vi "GeoData.vi"() -> ()   [LabVIEW 2017] (continued)
Niagara County\tH1\n14028\t36063\tBurt\tNY\tNiagara County\tH1\n14302\t36063\tNiagara falls\tNY\tNiagara County\tH1\n14032\t36063\tClarence center\tNY\tNiagara County\tH1\n14067\t36063\tGasport\tNY\tNiagara County\tH1\n14131\t36063\tRansomville\tNY\tNiagara County\tH1\n14008\t36063\tAppleton\tNY\tNiagara County\tH1\n14174\t36063\tYoungstown\tNY\tNiagara County\tH1\n14304\t36063\tNiagara falls\tNY\tNiagara County\tH1\n14012\t36063\tBarker\tNY\tNiagara County\tH1\n14108\t36063\tNewfane\tNY\tNiagara County\tH1\n14098\t36063\tLyndonville\tNY\tNiagara County\tH1\n14107\t36063\tModel city\tNY\tNiagara County\tH1\n14120\t36063\tNorth tonawanda\tNY\tNiagara County\tH1\n14001\t36063\tAkron\tNY\tNiagara County\tH1\n14092\t36063\tLewiston\tNY\tNiagara County\tH1\n14132\t36063\tSanborn\tNY\tNiagara County\tH1\n14303\t36063\tNiagara falls\tNY\tNiagara County\tH1\n14301\t36063\tNiagara falls\tNY\tNiagara County\tH1\n14305\t36063\tNiagara falls\tNY\tNiagara County\tH1\n14095\t36063\tLockport\tNY\tNiagara County\tH1\n14144\t36063\tStella niagara\tNY\tNiagara County\tH1\n13483\t36065\tWestdale\tNY\tOneida County\tH1\n13461\t36065\tSherrill\tNY\tOneida County\tH1\n13313\t36065\tBridgewater\tNY\tOneida County\tH1\n13301\t36065\tAlder creek\tNY\tOneida County\tH1\n13123\t36065\tNorth bay\tNY\tOneida County\tH1\n13338\t36065\tForestport\tNY\tOneida County\tH1\n13478\t36065\tVerona\tNY\tOneida County\tH1\n13354\t36065\tHolland patent\tNY\tOneida County\tH1\n13322\t36065\tClayville\tNY\tOneida County\tH1\n13486\t36065\tWesternville\tNY\tOneida County\tH1\n13032\t36065\tCanastota\tNY\tOneida County\tH1\n13308\t36065\tBlossvale\tNY\tOneida County\tH1\n13319\t36065\tChadwicks\tNY\tOneida County\tH1\n13413\t36065\tNew hartford\tNY\tOneida County\tH1\n13323\t36065\tClinton\tNY\tOneida County\tH1\n13501\t36065\tUtica\tNY\tOneida County\tH1\n13440\t36065\tRome\tNY\tOneida County\tH1\n13469\t36065\tStittville\tNY\tOneida County\tH1\n13441\t36065\tRome\tNY\tOneida County\tH1\n13162\t36065\tVerona beach\tNY\tOneida County\tH1\n13456\t36065\tSauquoit\tNY\tOneida County\tH1\n13495\t36065\tYorkville\tNY\tOneida County\tH1\n13424\t36065\tOriskany\tNY\tOneida County\tH1\n13362\t36065\tKnoxboro\tNY\tOneida County\tH1\n13304\t36065\tBarneveld\tNY\tOneida County\tH1\n13303\t36065\tAva\tNY\tOneida County\tH1\n13403\t36065\tMarcy\tNY\tOneida County\tH1\n13438\t36065\tRemsen\tNY\tOneida County\tH1\n13491\t36065\tWest winfield\tNY\tOneida County\tH1\n13417\t36065\tNew york mills\tNY\tOneida County\tH1\n13431\t36065\tPoland\tNY\tOneida County\tH1\n13435\t36065\tProspect\tNY\tOneida County\tH1\n13341\t36065\tFranklin springs\tNY\tOneida County\tH1\n13318\t36065\tCassville\tNY\tOneida County\tH1\n13409\t36065\tMunnsville\tNY\tOneida County\tH1\n13471\t36065\tTaberg\tNY\tOneida County\tH1\n13502\t36065\tUtica\tNY\tOneida County\tH1\n13490\t36065\tWestmoreland\tNY\tOneida County\tH1\n13321\t36065\tClark mills\tNY\tOneida County\tH1\n13401\t36065\tMc connellsville\tNY\tOneida County\tH1\n13042\t36065\tCleveland\tNY\tOneida County\tH1\n13309\t36065\tBoonville\tNY\tOneida County\tH1\n13316\t36065\tCamden\tNY\tOneida County\tH1\n13402\t36065\tMadison\tNY\tOneida County\tH1\n13476\t36065\tVernon\tNY\tOneida County\tH1\n13480\t36065\tWaterville\tNY\tOneida County\tH1\n13425\t36065\tOriskany falls\tNY\tOneida County\tH1\n13477\t36065\tVernon center\tNY\tOneida County\tH1\n13421\t36065\tOneida\tNY\tOneida County\tH1\n13492\t36065\tWhitesboro\tNY\tOneida County\tH1\n13489\t36065\tWest leyden\tNY\tOneida County\tH1\n13054\t36065\tDurhamville\tNY\tOneida County\tH1\n13157\t36065\tSylvan beach\tNY\tOneida County\tH1\n13363\t36065\tLee center\tNY\tOneida County\tH1\n13494\t36065\tWoodgate\tNY\tOneida County\tH1\n13328\t36065\tDeansboro\tNY\tOneida County\tH1\n13352\t36065\tHinckley\tNY\tOneida County\tH1\n13455\t36065\tSangerfield\tNY\tOneida County\tH1\n13479\t36065\tWashington mills\tNY\tOneida County\tH1\n13504\t36065\tUtica\tNY\tOneida County\tH1\n13035\t36067\tCazenovia\tNY\tOnondaga County\tH1\n13036\t36067\tCentral square\tNY\tOnondaga County\tH1\n13166\t36067\tWeedsport\tNY\tOnondaga County\tH1\n13020\t36067\tApulia station\tNY\tOnondaga County\tH1\n13120\t36067\tNedrow\tNY\tOnondaga County\tH1\n13206\t36067\tSyracuse\tNY\tOnondaga County\tH1\n13207\t36067\tSyracuse\tNY\tOnondaga County\tH1\n13244\t36067\tSyracuse\tNY\tOnondaga County\tH1\n13218\t36067\tSyracuse\tNY\tOnondaga County\tH1\n13290\t36067\tSyracuse\tNY\tOnondaga County\tH1\n13031\t36067\tCamillus\tNY\tOnondaga County\tH1\n13027\t36067\tBaldwinsville\tNY\tOnondaga County\tH1\n13069\t36067\tFulton\tNY\tOnondaga County\tH1\n13090\t36067\tLiverpool\tNY\tOnondaga County\tH1\n13152\t36067\tSkaneateles\tNY\tOnondaga County\tH1\n13112\t36067\tMemphis\tNY\tOnondaga County\tH1\n13030\t36067\tBridgeport\tNY\tOnondaga County\tH1\n13141\t36067\tPreble\tNY\tOnondaga County\tH1\n13153\t36067\tSkaneateles falls\tNY\tOnondaga County\tH1\n13029\t36067\tBrewerton\tNY\tOnondaga County\tH1\n13033\t36067\tCato\tNY\tOnondaga County\tH1\n13084\t36067\tLa fayette\tNY\tOnondaga County\tH1\n13080\t36067\tJordan\tNY\tOnondaga County\tH1\n13110\t36067\tMarietta\tNY\tOnondaga County\tH1\n13219\t36067\tSyracuse\tNY\tOnondaga County\tH1\n13224\t36067\tSyracuse\tNY\tOnondaga County\tH1\n13210\t36067\tSyracuse\tNY\tOnondaga County\tH1\n13235\t36067\tSyracuse\tNY\tOnondaga County\tH1\n13063\t36067\tFabius\tNY\tOnondaga County\tH1\n13217\t36067\tSyracuse\tNY\tOnondaga County\tH1\n13201\t36067\tSyracuse\tNY\tOnondaga County\tH1\n13225\t36067\tSyracuse\tNY\tOnondaga County\tH1\n13078\t36067\tJamesville\tNY\tOnondaga County\tH1\n13088\t36067\tLiverpool\tNY\tOnondaga County\tH1\n13077\t36067\tHomer\tNY\tOnondaga County\tH1\n13135\t36067\tPhoenix\tNY\tOnondaga County\tH1\n13108\t36067\tMarcellus\tNY\tOnondaga County\tH1\n13122\t36067\tNew woodstock\tNY\tOnondaga County\tH1\n13214\t36067\tSyracuse\tNY\tOnondaga County\tH1\n13215\t36067\tSyracuse\tNY\tOnondaga County\tH1\n13212\t36067\tSyracuse\tNY\tOnondaga County\tH1\n13204\t36067\tSyracuse\tNY\tOnondaga County\tH1\n13261\t36067\tSyracuse\tNY\tOnondaga County\tH1\n13039\t36067\tCicero\tNY\tOnondaga County\tH1\n13037\t36067\tChittenango\tNY\tOnondaga County\tH1\n13104\t36067\tManlius\tNY\tOnondaga County\tH1\n13057\t36067\tEast syracuse\tNY\tOnondaga County\tH1\n13052\t36067\tDe ruyter\tNY\tOnondaga County\tH1\n13060\t36067\tElbridge\tNY\tOnondaga County\tH1\n13205\t36067\tSyracuse\tNY\tOnondaga County\tH1\n13089\t36067\tLiverpool\tNY\tOnondaga County\tH1\n13138\t36067\tPompey\tNY\tOnondaga County\tH1\n13051\t36067\tDelphi falls\tNY\tOnondaga County\tH1\n13119\t36067\tMottville\tNY\tOnondaga County\tH1\n13252\t36067\tSyracuse\tNY\tOnondaga County\tH1\n13021\t36067\tAuburn\tNY\tOnondaga County\tH1\n13202\t36067\tSyracuse\tNY\tOnondaga County\tH1\n13203\t36067\tSyracuse\tNY\tOnondaga County\tH1\n13116\t36067\tMinoa\tNY\tOnondaga County\tH1\n13137\t36067\tPlainville\tNY\tOnondaga County\tH1\n13082\t36067\tKirkville\tNY\tOnondaga County\tH1\n13066\t36067\tFayetteville\tNY\tOnondaga County\tH1\n13158\t36067\tTruxton\tNY\tOnondaga County\tH1\n13159\t36067\tTully\tNY\tOnondaga County\tH1\n13164\t36067\tWarners\tNY\tOnondaga County\tH1\n13208\t36067\tSyracuse\tNY\tOnondaga County\tH1\n13211\t36067\tSyracuse\tNY\tOnondaga County\tH1\n13209\t36067\tSyracuse\tNY\tOnondaga County\tH1\n13220\t36067\tSyracuse\tNY\tOnondaga County\tH1\n13041\t36067\tClay\tNY\tOnondaga County\tH1\n14512\t36069\tNaples\tNY\tOntario County\tH1\n14585\t36069\tWest bloomfield\tNY\tOntario County\tH1\n14534\t36069\tPittsford\tNY\tOntario County\tH1\n14472\t36069\tHoneoye falls\tNY\tOntario County\tH1\n14544\t36069\tRushville\tNY\tOntario County\tH1\n14425\t36069\tFarmington\tNY\tOntario County\tH1\n14463\t36069\tHall\tNY\tOntario County\tH1\n14475\t36069\tIonia\tNY\tOntario County\tH1\n14547\t36069\tSeneca castle\tNY\tOntario County\tH1\n14560\t36069\tSpringwater\tNY\tOntario County\tH1\n14424\t36069\tCanandaigua\tNY\tOntario County\tH1\n14504\t36069\tManchester\tNY\tOntario County\tH1\n14537\t36069\tPort gibson\tNY\tOntario County\tH1\n14485\t36069\tLima\tNY\tOntario County\tH1\n14487\t36069\tLivonia\tNY\tOntario County\tH1\n14513\t36069\tNewark\tNY\tOntario County\tH1\n14564\t36069\tVictor\tNY\tOntario County\tH1\n14561\t36069\tStanley\tNY\tOntario County\tH1\n14466\t36069\tHemlock\tNY\tOntario County\tH1\n14461\t36069\tGorham\tNY\tOntario County\tH1\n14432\t36069\tClifton springs\tNY\tOntario County\tH1\n14489\t36069\tLyons\tNY\tOntario County\tH1\n14456\t36069\tGeneva\tNY\tOntario County\tH1\n14471\t36069\tHoneoye\tNY\tOntario County\tH1\n14522\t36069\tPalmyra\tNY\tOntario County\tH1\n14548\t36069\tShortsville\tNY\tOntario County\tH1\n14453\t36069\tFishers\tNY\tOntario County\tH1\n14518\t36069\tOaks corners\tNY\tOntario County\tH1\n14469\t36069\tBloomfield\tNY\tOntario County\tH1\n14532\t36069\tPhelps\tNY\tOntario County\tH1\n10924\t36071\tGoshen\tNY\tOrange County\tH1\n10987\t36071\tTuxedo park\tNY\tOrange County\tH1\n12520\t36071\tCornwall on hudson\tNY\tOrange County\tH1\n12553\t36071\tNew windsor\tNY\tOrange County\tH1\n12566\t36071\tPine bush\tNY\tOrange County\tH1\n12589\t36071\tWallkill\tNY\tOrange County\tH1\n12575\t36071\tRock tavern\tNY\tOrange County\tH1\n12785\t36071\tWestbrookville\tNY\tOrange County\tH1\n10910\t36071\tArden\tNY\tOrange County\tH1\n10918\t36071\tChester\tNY\tOrange County\tH1\n12543\t36071\tMaybrook\tNY\tOrange County\tH1\n12586\t36071\tWalden\tNY\tOrange County\tH1\n10933\t36071\tJohnson\tNY\tOrange County\tH1\n10981\t36071\tSugar loaf\tNY\tOrange County\tH1\n10979\t36071\tSterling forest\tNY\tOrange County\tH1\n10959\t36071\tNew milford\tNY\tOrange County\tH1\n10925\t36071\tGreenwood lake\tNY\tOrange County\tH1\n10958\t36071\tNew hampton\tNY\tOrange County\tH1\n10985\t36071\tThompson ridge\tNY\tOrange County\tH1\n12518\t36071\tCornwall\tNY\tOrange County\tH1\n10928\t36071\tHighland falls\tNY\tOrange County\tH1\n10919\t36071\tCircleville\tNY\tOrange County\tH1\n12551\t36071\tNewburgh\tNY\tOrange County\tH1\n12584\t36071\tVails gate\tNY\tOrange County\tH1\n10953\t36071\tMountainville\tNY\tOrange County\tH1\n10914\t36071\tBlooming grove\tNY\tOrange County\tH1\n12549\t36071\tMontgomery\tNY\tOrange County\tH1\n12577\t36071\tSalisbury mills\tNY\tOrange County\tH1\n12729\t36071\tCuddebackville\tNY\tOrange County\tH1\n10932\t36071\tHowells\tNY\tOrange County\tH1\n10917\t36071\tCentral valley\tNY\tOrange County\tH1\n10926\t36071\tHarriman\tNY\tOrange County\tH1\n10998\t36071\tWesttown\tNY\tOrange County\tH1\n12542\t36071\tMarlboro\tNY\tOrange County\tH1\n12721\t36071\tBloomingburg\tNY\tOrange County\tH1\n10916\t36071\tCampbell hall\tNY\tOrange County\tH1\n10988\t36071\tUnionville\tNY\tOrange County\tH1\n10975\t36071\tSouthfields\tNY\tOrange County\tH1\n10940\t36071\tMiddletown\tNY\tOrange County\tH1\n10950\t36071\tMonroe\tNY\tOrange County\tH1\n12754\t36071\tLiberty\tNY\tOrange County\tH1\n10912\t36071\tBellvale\tNY\tOrange County\tH1\n10915\t36071\tBullville\tNY\tOrange County\tH1\n10941\t36071\tMiddletown\tNY\tOrange County\tH1\n10930\t36071\tHighland mills\tNY\tOrange County\tH1\n10990\t36071\tWarwick\tNY\tOrange County\tH1\n10973\t36071\tSlate hill\tNY\tOrange County\tH1\n10969\t36071\tPine island\tNY\tOrange County\tH1\n10996\t36071\tWest point\tNY\tOrange County\tH1\n12771\t36071\tPort jervis\tNY\tOrange County\tH1\n12552\t36071\tNewburgh\tNY\tOrange County\tH1\n12555\t36071\tNewburgh\tNY\tOrange County\tH1\n10921\t36071\tFlorida\tNY\tOrange County\tH1\n10963\t36071\tOtisville\tNY\tOrange County\tH1\n10992\t36071\tWashingtonville\tNY\tOrange County\tH1\n12550\t36071\tNewburgh\tNY\tOrange County\tH1\n12780\t36071\tSparrow bush\tNY\tOrange County\tH1\n10949\t36071\tMonroe\tNY\tOrange County\tH1\n12746\t36071\tHuguenot\tNY\tOrange County\tH1\n10922\t36071\tFort montgomery\tNY\tOrange County\tH1\n14464\t36073\tHamlin\tNY\tOrleans County\tH1\n14476\t36073\tKendall\tNY\tOrleans County\tH1\n14452\t36073\tFancher\tNY\tOrleans County\tH1\n14105\t36073\tMiddleport\tNY\tOrleans County\tH1\n14420\t36073\tBrockport\tNY\tOrleans County\tH1\n14416\t36073\tBergen\tNY\tOrleans County\tH1\n14058\t36073\tElba\tNY\tOrleans County\tH1\n14422\t36073\tByron\tNY\tOrleans County\tH1\n14429\t36073\tClarendon\tNY\tOrleans County\tH1\n14012\t36073\tBarker\tNY\tOrleans County\tH1\n14103\t36073\tMedina\tNY\tOrleans County\tH1\n14098\t36073\tLyndonville\tNY\tOrleans County\tH1\n14477\t36073\tKent\tNY\tOrleans County\tH1\n14125\t36073\tOakfield\tNY\tOrleans County\tH1\n14411\t36073\tAlbion\tNY\tOrleans County\tH1\n14470\t36073\tHolley\tNY\tOrleans County\tH1\n14571\t36073\tWaterport\tNY\tOrleans County\tH1\n14479\t36073\tKnowlesville\tNY\tOrleans County\tH1\n13036\t36075\tCentral square\tNY\tOswego County\tH1\n13074\t36075\tHannibal\tNY\tOswego County\tH1\n13111\t36075\tMartville\tNY\tOswego County\tH1\n13145\t36075\tSandy creek\tNY\tOswego County\tH1\n13302\t36075\tAltmar\tNY\tOswego County\tH1\n13483\t36075\tWestdale\tNY\tOswego County\tH1\n13144\t36075\tRichland\tNY\tOswego County\tH1\n13167\t36075\tWest monroe\tNY\tOswego County\tH1\n13132\t36075\tPennellville\tNY\tOswego County\tH1\n13069\t36075\tFulton\tNY\tOswego County\tH1\n13121\t36075\tNew haven\tNY\tOswego County\tH1\n13033\t36075\tCato\tNY\tOswego County\tH1\n13493\t36075\tWilliamstown\tNY\tOswego County\tH1\n13661\t36075\tMannsville\tNY\tOswego County\tH1\n13426\t36075\tOrwell\tNY\tOswego County\tH1\n13093\t36075\tLycoming\tNY\tOswego County\tH1\n13044\t36075\tConstantia\tNY\tOswego County\tH1\n13142\t36075\tPulaski\tNY\tOswego County\tH1\n13135\t36075\tPhoenix\tNY\tOswego County\tH1\n13103\t36075\tMallory\tNY\tOswego County\tH1\n13437\t36075\tRedfield\tNY\tOswego County\tH1\n13126\t36075\tOswego\tNY\tOswego County\tH1\n13042\t36075\tCleveland\tNY\tOswego County\tH1\n13156\t36075\tSterling\tNY\tOswego County\tH1\n13316\t36075\tCamden\tNY\tOswego County\tH1\n13076\t36075\tHastings\tNY\tOswego County\tH1\n13115\t36075\tMinetto\tNY\tOswego County\tH1\n13114\t36075\tMexico\tNY\tOswego County\tH1\n13131\t36075\tParish\tNY\tOswego County\tH1\n13028\t36075\tBernhards bay\tNY\tOswego County\tH1\n13083\t36075\tLacona\tNY\tOswego County\tH1\n12155\t36077\tSchenevus\tNY\tOtsego County\tH1\n13796\t36077\tLaurens\tNY\tOtsego County\tH1\n13315\t36077\tBurlington flats\tNY\tOtsego County\tH1\n13333\t36077\tEast springfield\tNY\tOtsego County\tH1\n13457\t36077\tSchuyler lake\tNY\tOtsego County\tH1\n12149\t36077\tRichmondville\tNY\tOtsego County\tH1\n13320\t36077\tCherry valley\tNY\tOtsego County\tH1\n13450\t36077\tRoseboom\tNY\tOtsego County\tH1\n13834\t36077\tPortlandville\tNY\tOtsego County\tH1\n13459\t36077\tSharon springs\tNY\tOtsego County\tH1\n13849\t36077\tUnadilla\tNY\tOtsego County\tH1\n13361\t36077\tJordanville\tNY\tOtsego County\tH1\n13482\t36077\tWest burlington\tNY\tOtsego County\tH1\n13415\t36077\tNew lisbon\tNY\tOtsego County\tH1\n12036\t36077\tCharlotteville\tNY\tOtsego County\tH1\n13335\t36077\tEdmeston\tNY\tOtsego County\tH1\n13809\t36077\tMount upton\tNY\tOtsego County\tH1\n13337\t36077\tFly creek\tNY\tOtsego County\tH1\n12043\t36077\tCobleskill\tNY\tOtsego County\tH1\n13348\t36077\tHartwick\tNY\tOtsego County\tH1\n13317\t36077\tCanajoharie\tNY\tOtsego County\tH1\n13411\t36077\tNew berlin\tNY\tOtsego County\tH1\n13491\t36077\tWest winfield\tNY\tOtsego County\tH1\n13485\t36077\tWest edmeston\tNY\tOtsego County\tH1\n13439\t36077\tRichfield springs\tNY\tOtsego County\tH1\n13733\t36077\tBainbridge\tNY\tOtsego County\tH1\n13810\t36077\tMount vision\tNY\tOtsego County\tH1\n13861\t36077\tWest oneonta\tNY\tOtsego County\tH1\n13825\t36077\tOtego\tNY\tOtsego County\tH1\n13488\t36077\tWestford\tNY\tOtsego County\tH1\n12064\t36077\tEast worcester\tNY\tOtsego County\tH1\n13747\t36077\tColliersville\tNY\tOtsego County\tH1\n13838\t36077\tSidney\tNY\tOtsego County\tH1\n13326\t36077\tCooperstown\tNY\tOtsego County\tH1\n13807\t36077\tMilford\tNY\tOtsego County\tH1\n13468\t36077\tSpringfield center\tNY\tOtsego County\tH1\n13750\t36077\tDavenport\tNY\tOtsego County\tH1\n13776\t36077\tGilbertsville\tNY\tOtsego County\tH1\n12116\t36077\tMaryland\tNY\tOtsego County\tH1\n12197\t36077\tWorcester\tNY\tOtsego County\tH1\n13820\t36077\tOneonta\tNY\tOtsego County\tH1\n13808\t36077\tMorris\tNY\tOtsego County\tH1\n13775\t36077\tFranklin\tNY\tOtsego County\tH1\n13843\t36077\tSouth new berlin\tNY\tOtsego County\tH1\n13859\t36077\tWells bridge\tNY\tOtsego County\tH1\n13342\t36077\tGarrattsville\tNY\tOtsego County\tH1\n12533\t36079\tHopewell junction\tNY\tPutnam County\tH1\n12563\t36079\tPatterson\tNY\tPutnam County\tH1\n10542\t36079\tMahopac falls\tNY\tPutnam County\tH1\n10512\t36079\tCarmel\tNY\tPutnam County\tH1\n10509\t36079\tBrewster\tNY\tPutnam County\tH1\n12564\t36079\tPawling\tNY\tPutnam County\tH1\n10505\t36079\tBaldwin place\tNY\tPutnam County\tH1\n10516\t36079\tCold spring\tNY\tPutnam County\tH1\n12531\t36079\tHolmes\tNY\tPutnam County\tH1\n10541\t36079\tMahopac\tNY\tPutnam County\tH1\n10579\t36079\tPutnam valley\tNY\tPutnam County\tH1\n12582\t36079\tStormville\tNY\tPutnam County\tH1\n10524\t36079\tGarrison\tNY\tPutnam County\tH1\n10588\t36079\tShrub oak\tNY\tPutnam County\tH1\n10567\t36079\tCortlandt manor\tNY\tPutnam County\tH1\n10598\t36079\tYorktown heights\tNY\tPutnam County\tH1\n12524\t36079\tFishkill\tNY\tPutnam County\tH1\n10537\t36079\tLake peekskill\tNY\tPutnam County\tH1\n11001\t36081\tFloral park\tNY\tQueens County\tH6\n11102\t36081\tAstoria\tNY\tQueens County\tH6\n11369\t36081\tEast elmhurst\tNY\tQueens County\tH6\n11418\t36081\tRichmond hill\tNY\tQueens County\tH6\n11420\t36081\tSouth ozone park\tNY\tQueens County\tH6\n11422\t36081\tRosedale\tNY\tQueens County\tH6\n11419\t36081\tSouth richmond hill\tNY\tQueens County\tH6\n11427\t36081\tQueens village\tNY\tQueens County\tH6\n11693\t36081\tFar rockaway\tNY\tQueens County\tH6\n11020\t36081\tGreat neck\tNY\tQueens County\tH6\n11106\t36081\tAstoria\tNY\tQueens County\tH6\n11354\t36081\tFlushing\tNY\tQueens County\tH6\n11368\t36081\tCorona\tNY\tQueens County\tH6\n11370\t36081\tEast elmhurst\tNY\tQueens County\tH6\n11372\t36081\tJackson heights\tNY\tQueens County\tH6\n11377\t36081\tWoodside\tNY\tQueens County\tH6\n11413\t36081\tSpringfield gardens\tNY\tQueens County\tH6\n11433\t36081\tJamaica\tNY\tQueens County\tH6\n11417\t36081\tOzone park\tNY\tQueens County\tH6\n11428\t36081\tQueens village\tNY\tQueens County\tH6\n11692\t36081\tArverne\tNY\tQueens County\tH6\n11371\t36081\tFlushing\tNY\tQueens County\tH6\n11359\t36081\tBayside\tNY\tQueens County\tH6\n11208\t36081\tBrooklyn\tNY\tQueens County\tH6\n11352\t36081\tFlushing\tNY\tQueens County\tH6\n11366\t36081\tFresh meadows\tNY\tQueens County\tH6\n11430\t36081\tJamaica\tNY\tQueens County\tH6\n11439\t36081\tJamaica\tNY\tQueens County\tH6\n11431\t36081\tJamaica\tNY\tQueens County\tH6\n11405\t36081\tJamaica\tNY\tQueens County\tH6\n11105\t36081\tAstoria\tNY\tQueens County\tH6\n11109\t36081\tLong island city\tNY\tQueens County\tH6\n11367\t36081\tFlushing\tNY\tQueens County\tH6\n11360\t36081\tBayside\tNY\tQueens County\tH6\n11412\t36081\tSaint albans\tNY\tQueens County\tH6\n11414\t36081\tHoward beach\tNY\tQueens County\tH6\n11423\t36081\tHollis\tNY\tQueens County\tH6\n11691\t36081\tFar rockaway\tNY\tQueens County\tH6\n11580\t36081\tValley stream\tNY\tQueens County\tH6\n11386\t36081\tRidgewood\tNY\tQueens County\tH6\n11101\t36081\tLong island city\tNY\tQueens County\tH6\n11103\t36081\tAstoria\tNY\tQueens County\tH6\n11362\t36081\tLittle neck\tNY\tQueens County\tH6\n11358\t36081\tFlushing\tNY\tQueens County\tH6\n11379\t36081\tMiddle village\tNY\tQueens County\tH6\n11411\t36081\tCambria heights\tNY\tQueens County\tH6\n11435\t36081\tJamaica\tNY\tQueens County\tH6\n11429\t36081\tQueens village\tNY\tQueens County\tH6\n11436\t36081\tJamaica\tNY\tQueens County\tH6\n11697\t36081\tBreezy point\tNY\tQueens County\tH6\n11559\t36081\tLawrence\tNY\tQueens County\tH6\n11351\t36081\tFlushing\tNY\tQueens County\tH6\n11004\t36081\tGlen oaks\tNY\tQueens County\tH6\n11104\t36081\tSunnyside\tNY\tQueens County\tH6\n11355\t36081\tFlushing\tNY\tQueens County\tH6\n11357\t36081\tWhitestone\tNY\tQueens County\tH6\n11361\t36081\tBayside\tNY\tQueens County\tH6\n11356\t36081\tCollege point\tNY\tQueens County\tH6\n11374\t36081\tRego park\tNY\tQueens County\tH6\n11385\t36081\tRidgewood\tNY\tQueens County\tH6\n11378\t36081\tMaspeth\tNY\tQueens County\tH6\n11415\t36081\tKew gardens\tNY\tQueens County\tH6\n11434\t36081\tJamaica\tNY\tQueens County\tH6\n11694\t36081\tRockaway park\tNY\tQueens County\tH6\n11005\t36081\tFloral park\tNY\tQueens County\tH6\n11380\t36081\tElmhurst\tNY\tQueens County\tH6\n11381\t36081\tFlushing\tNY\tQueens County\tH6\n11040\t36081\tNew hyde park\tNY\tQueens County\tH6\n11364\t36081\tOakland gardens\tNY\tQueens County\tH6\n11375\t36081\tForest hills\tNY\tQueens County\tH6\n11421\t36081\tWoodhaven\tNY\tQueens County\tH6\n11424\t36081\tJamaica\tNY\tQueens County\tH6\n11499\t36081\tJamaica\tNY\tQueens County\tH6\n11425\t36081\tJamaica\tNY\tQueens County\tH6\n11365\t36081\tFresh meadows\tNY\tQueens County\tH6\n11363\t36081\tLittle neck\tNY\tQueens County\tH6\n11373\t36081\tElmhurst\tNY\tQueens County\tH6\n11416\t36081\tOzone park\tNY\tQueens County\tH6\n11432\t36081\tJamaica\tNY\tQueens County\tH6\n11426\t36081\tBellerose\tNY\tQueens County\tH6\n11451\t36081\tJamaica\tNY\tQueens County\tH6\n12169\t36083\tStephentown\tNY\tRensselaer County\tH1\n12052\t36083\tCropseyville\tNY\tRensselaer County\tH1\n12089\t36083\tHoosick\tNY\tRensselaer County\tH1\n12018\t36083\tAverill park\tNY\tRensselaer County\tH1\n12144\t36083\tRensselaer\tNY\tRensselaer County\tH1\n12185\t36083\tValley falls\tNY\tRensselaer County\tH1\n12153\t36083\tSand lake\tNY\tRensselaer County\tH1\n12028\t36083\tBuskirk\tNY\tRensselaer County\tH1\n12094\t36083\tJohnsonville\tNY\tRensselaer County\tH1\n12118\t36083\tMechanicville\tNY\tRensselaer County\tH1\n12182\t36083\tTroy\tNY\tRensselaer County\tH1\n12184\t36083\tValatie\tNY\tRensselaer County\tH1\n12168\t36083\tStephentown\tNY\tRensselaer County\tH1\n12121\t36083\tMelrose\tNY\tRensselaer County\tH1\n12057\t36083\tEagle bridge\tNY\tRensselaer County\tH1\n12040\t36083\tCherry plain\tNY\tRensselaer County\tH1\n12033\t36083\tCastleton on hudson\tNY\tRensselaer County\tH1\n12061\t36083\tEast greenbush\tNY\tRensselaer County\tH1\n12123\t36083\tNassau\tNY\tRensselaer County\tH1\n12140\t36083\tPoestenkill\tNY\tRensselaer County\tH1\n12090\t36083\tHoosick falls\tNY\tRensselaer County\tH1\n12062\t36083\tEast nassau\tNY\tRensselaer County\tH1\n12138\t36083\tPetersburg\tNY\tRensselaer County\tH1\n12180\t36083\tTroy\tNY\tRensselaer County\tH1\n12198\t36083\tWynantskill\tNY\tRensselaer County\tH1\n12022\t36083\tBerlin\tNY\tRensselaer County\tH1\n12082\t36083\tGrafton\tNY\tRensselaer County\tH1\n12156\t36083\tSchodack landing\tNY\tRensselaer County\tH1\n12154\t36083\tSchaghticoke\tNY\tRensselaer County\tH1\n12196\t36083\tWest sand lake\tNY\tRensselaer County\tH1\n12181\t36083\tTroy\tNY\tRensselaer County\tH1\n12024\t36083\tBrainard\tNY\tRensselaer County\tH1\n12063\t36083\tEast schodack\tNY\tRensselaer County\tH1\n12133\t36083\tNorth hoosick\tNY\tRensselaer County\tH1\n10301\t36085\tStaten island\tNY\tRichmond County\tH6\n10312\t36085\tStaten island\tNY\tRichmond County\tH6\n10308\t36085\tStaten island\tNY\tRichmond County\tH6\n10303\t36085\tStaten island\tNY\tRichmond County\tH6\n10313\t36085\tStaten island\tNY\tRichmond County\tH6\n10302\t36085\tStaten island\tNY\tRichmond County\tH6\n10310\t36085\tStaten island\tNY\tRichmond County\tH6\n10306\t36085\tStaten island\tNY\tRichmond County\tH6\n10309\t36085\tStaten island\tNY\tRichmond County\tH6\n10307\t36085\tStaten island\tNY\tRichmond County\tH6\n10314\t36085\tStaten island\tNY\tRichmond County\tH6\n10311\t36085\tStaten island\tNY\tRichmond County\tH6\n10304\t36085\tStaten island\tNY\tRichmond County\tH6\n10305\t36085\tStaten island\tNY\tRichmond County\tH6\n10901\t36087\tSuffern\tNY\tRockland County\tH1\n10954\t36087\tNanuet\tNY\tRockland County\tH1\n10989\t36087\tValley cottage\tNY\tRockland County\tH1\n10968\t36087\tPiermont\tNY\tRockland County\tH1\n10994\t36087\tWest nyack\tNY\tRockland County\tH1\n10976\t36087\tSparkill\tNY\tRockland County\tH1\n10923\t36087\tGarnerville\tNY\tRockland County\tH1\n10982\t36087\tTallman\tNY\tRockland County\tH1\n10913\t36087\tBlauvelt\tNY\tRockland County\tH1\n10970\t36087\tPomona\tNY\tRockland County\tH1\n10964\t36087\tPalisades\tNY\tRockland County\tH1\n10977\t36087\tSpring valley\tNY\tRockland County\tH1\n10952\t36087\tMonsey\tNY\tRockland County\tH1\n10965\t36087\tPearl river\tNY\tRockland County\tH1\n10993\t36087\tWest haverstraw\tNY\tRockland County\tH1\n10984\t36087\tThiells\tNY\tRockland County\tH1\n10983\t36087\tTappan\tNY\tRockland County\tH1\n10962\t36087\tOrangeburg\tNY\tRockland County\tH1\n10956\t36087\tNew city\tNY\tRockland County\tH1\n10927\t36087\tHaverstraw\tNY\tRockland County\tH1\n10960\t36087\tNyack\tNY\tRockland County\tH1\n10980\t36087\tStony point\tNY\tRockland County\tH1\n10974\t36087\tSloatsburg\tNY\tRockland County\tH1\n10911\t36087\tBear mountain\tNY\tRockland County\tH1\n10920\t36087\tCongers\tNY\tRockland County\tH1\n10986\t36087\tTomkins cove\tNY\tRockland County\tH1\n10931\t36087\tHillburn\tNY\tRockland County\tH1\n13676\t36089\tPotsdam\tNY\tSt. Lawrence County\tH1\n13677\t36089\tPyrites\tNY\tSt. Lawrence County\tH1\n13623\t36089\tChippewa bay\tNY\tSt. Lawrence County\tH1\n12980\t36089\tSaint regis falls\tNY\tSt. Lawrence County\tH1\n13617\t36089\tCanton\tNY\tSt. Lawrence County\tH1\n13669\t36089\tOgdensburg\tNY\tSt. Lawrence County\tH1\n13684\t36089\tRussell\tNY\tSt. Lawrence County\tH1\n13691\t36089\tTheresa\tNY\tSt. Lawrence County\tH1\n13613\t36089\tBrasher falls\tNY\tSt. Lawrence County\tH1\n12967\t36089\tNorth lawrence\tNY\tSt. Lawrence County\tH1\n13666\t36089\tNewton falls\tNY\tSt. Lawrence County\tH1\n12922\t36089\tChildwold\tNY\tSt. Lawrence County\tH1\n13645\t36089\tHailesboro\tNY\tSt. Lawrence County\tH1\n12914\t36089\tBombay\tNY\tSt. Lawrence County\tH1\n13668\t36089\tNorwood\tNY\tSt. Lawrence County\tH1\n13662\t36089\tMassena\tNY\tSt. Lawrence County\tH1\n13660\t36089\tMadrid\tNY\tSt. Lawrence County\tH1\n13690\t36089\tStar lake\tNY\tSt. Lawrence County\tH1\n12965\t36089\tNicholville\tNY\tSt. Lawrence County\tH1\n13681\t36089\tRichville\tNY\tSt. Lawrence County\tH1\n13694\t36089\tWaddington\tNY\tSt. Lawrence County\tH1\n13658\t36089\tLisbon\tNY\tSt. Lawrence County\tH1\n13672\t36089\tParishville\tNY\tSt. Lawrence County\tH1\n13696\t36089\tWest stockholm\tNY\tSt. Lawrence County\tH1\n13633\t36089\tDe peyster\tNY\tSt. Lawrence County\tH1\n13654\t36089\tHeuvelton\tNY\tSt. Lawrence County\tH1\n13635\t36089\tEdwards\tNY\tSt. Lawrence County\tH1\n13648\t36089\tHarrisville\tNY\tSt. Lawrence County\tH1\n13647\t36089\tHannawa falls\tNY\tSt. Lawrence County\tH1\n13630\t36089\tDe kalb junction\tNY\tSt. Lawrence County\tH1\n13608\t36089\tAntwerp\tNY\tSt. Lawrence County\tH1\n13667\t36089\tNorfolk\tNY\tSt. Lawrence County\tH1\n13680\t36089\tRensselaer falls\tNY\tSt. Lawrence County\tH1\n13646\t36089\tHammond\tNY\tSt. Lawrence County\tH1\n13652\t36089\tHermon\tNY\tSt. Lawrence County\tH1\n12927\t36089\tCranberry lake\tNY\tSt. Lawrence County\tH1\n12949\t36089\tLawrenceville\tNY\tSt. Lawrence County\tH1\n12973\t36089\tPiercefield\tNY\tSt. Lawrence County\tH1\n13625\t36089\tColton\tNY\tSt. Lawrence County\tH1\n13695\t36089\tWanakena\tNY\tSt. Lawrence County\tH1\n13614\t36089\tBrier hill\tNY\tSt. Lawrence County\tH1\n13664\t36089\tMorristown\tNY\tSt. Lawrence County\tH1\n13670\t36089\tOswegatchie\tNY\tSt. Lawrence County\tH1\n12930\t36089\tDickinson center\tNY\tSt. Lawrence County\tH1\n12986\t36089\tTupper lake\tNY\tSt. Lawrence County\tH1\n13642\t36089\tGouverneur\tNY\tSt. Lawrence County\tH1\n13621\t36089\tChase mills\tNY\tSt. Lawrence County\tH1\n13687\t36089\tSouth colton\tNY\tSt. Lawrence County\tH1\n13679\t36089\tRedwood\tNY\tSt. Lawrence County\tH1\n13697\t36089\tWinthrop\tNY\tSt. Lawrence County\tH1\n13649\t36089\tHelena\tNY\tSt. Lawrence County\tH1\n13639\t36089\tFine\tNY\tSt. Lawrence County\tH1\n13699\t36089\tPotsdam\tNY\tSt. Lawrence County\tH1\n13678\t36089\tRaymondville\tNY\tSt. Lawrence County\tH1\n12828\t36091\tFort edward\tNY\tSaratoga County\tH1\n12833\t36091\tGreenfield center\tNY\tSaratoga County\tH1\n12884\t36091\tVictory mills\tNY\tSaratoga County\tH1\n12019\t36091\tBallston lake\tNY\tSaratoga County\tH1\n12086\t36091\tHagaman\tNY\tSaratoga County\tH1\n12871\t36091\tSchuylerville\tNY\tSaratoga County\tH1\n12010\t36091\tAmsterdam\tNY\tSaratoga County\tH1\n12074\t36091\tGalway\tNY\tSaratoga County\tH1\n12118\t36091\tMechanicville\tNY\tSaratoga County\tH1\n12302\t36091\tSchenectady\tNY\tSaratoga County\tH1\n12866\t36091\tSaratoga springs\tNY\tSaratoga County\tH1\n12831\t36091\tGansevoort\tNY\tSaratoga County\tH1\n12835\t36091\tHadley\tNY\tSaratoga County\tH1\n12188\t36091\tWaterford\tNY\tSaratoga County\tH1\n12020\t36091\tBallston spa\tNY\tSaratoga County\tH1\n12025\t36091\tBroadalbin\tNY\tSaratoga County\tH1\n12850\t36091\tMiddle grove\tNY\tSaratoga County\tH1\n12859\t36091\tPorter corners\tNY\tSaratoga County\tH1\n12027\t36091\tBurnt hills\tNY\tSaratoga County\tH1\n12822\t36091\tCorinth\tNY\tSaratoga County\tH1\n12151\t36091\tRound lake\tNY\tSaratoga County\tH1\n12148\t36091\tRexford\tNY\tSaratoga County\tH1\n12170\t36091\tStillwater\tNY\tSaratoga County\tH1\n12065\t36091\tClifton park\tNY\tSaratoga County\tH1\n12803\t36091\tSouth glens falls\tNY\tSaratoga County\tH1\n12134\t36091\tNorthville\tNY\tSaratoga County\tH1\n12863\t36091\tRock city falls\tNY\tSaratoga County\tH1\n12305\t36093\tSchenectady\tNY\tSchenectady County\tH1\n12019\t36093\tBallston lake\tNY\tSchenectady County\tH1\n12157\t36093\tSchoharie\tNY\tSchenectady County\tH1\n12137\t36093\tPattersonville\tNY\tSchenectady County\tH1\n12010\t36093\tAmsterdam\tNY\tSchenectady County\tH1\n12053\t36093\tDelanson\tNY\tSchenectady County\tH1\n12056\t36093\tDuanesburg\tNY\tSchenectady County\tH1\n12302\t36093\tSchenectady\tNY\tSchenectady County\tH1\n12306\t36093\tSchenectady\tNY\tSchenectady County\tH1\n12066\t36093\tEsperance\tNY\tSchenectady County\tH1\n12309\t36093\tSchenectady\tNY\tSchenectady County\tH1\n12027\t36093\tBurnt hills\tNY\tSchenectady County\tH1\n12303\t36093\tSchenectady\tNY\tSchenectady County\tH1\n12304\t36093\tSchenectady\tNY\tSchenectady County\tH1\n12150\t36093\tRotterdam junction\tNY\tSchenectady County\tH1\n12345\t36093\tSchenectady\tNY\tSchenectady County\tH1\n12141\t36093\tQuaker street\tNY\tSchenectady County\tH1\n12009\t36093\tAltamont\tNY\tSchenectady County\tH1\n12301\t36093\tSchenectady\tNY\tSchenectady County\tH1\n12008\t36093\tAlplaus\tNY\tSchenectady County\tH1\n12308\t36093\tSchenectady\tNY\tSchenectady County\tH1\n12307\t36093\tSchenectady\tNY\tSchenectady County\tH1\n12175\t36095\tSummit\tNY\tSchoharie County\tH1\n12194\t36095\tWest fulton\tNY\tSchoharie County\tH1\n12469\t36095\tPreston hollow\tNY\tSchoharie County\tH1\n12149\t36095\tRichmondville\tNY\tSchoharie County\tH1\n12157\t36095\tSchoharie\tNY\tSchoharie County\tH1\n12167\t36095\tStamford\tNY\tSchoharie County\tH1\n13320\t36095\tCherry valley\tNY\tSchoharie County\tH1\n12131\t36095\tNorth blenheim\tNY\tSchoharie County\tH1\n12035\t36095\tCentral bridge\tNY\tSchoharie County\tH1\n12023\t36095\tBerne\tNY\tSchoharie County\tH1\n12053\t36095\tDelanson\tNY\tSchoharie County\tH1\n12093\t36095\tJefferson\tNY\tSchoharie County\tH1\n12122\t36095\tMiddleburgh\tNY\tSchoharie County\tH1\n13459\t36095\tSharon springs\tNY\tSchoharie County\tH1\n12160\t36095\tSloansville\tNY\tSchoharie County\tH1\n12036\t36095\tCharlotteville\tNY\tSchoharie County\tH1\n12092\t36095\tHowes cave\tNY\tSchoharie County\tH1\n12066\t36095\tEsperance\tNY\tSchoharie County\tH1\n12071\t36095\tFultonham\tNY\tSchoharie County\tH1\n12073\t36095\tGallupville\tNY\tSchoharie County\tH1\n12043\t36095\tCobleskill\tNY\tSchoharie County\tH1\n12166\t36095\tSprakers\tNY\tSchoharie County\tH1\n12064\t36095\tEast worcester\tNY\tSchoharie County\tH1\n12076\t36095\tGilboa\tNY\tSchoharie County\tH1\n12187\t36095\tWarnerville\tNY\tSchoharie County\tH1\n12031\t36095\tCarlisle\tNY\tSchoharie County\tH1\n14824\t36097\tCayuta\tNY\tSchuyler County\tH1\n14887\t36097\tTyrone\tNY\tSchuyler County\tH1\n14812\t36097\tBeaver dams\tNY\tSchuyler County\tH1\n14837\t36097\tDundee\tNY\tSchuyler County\tH1\n14889\t36097\tVan etten\tNY\tSchuyler County\tH1\n14867\t36097\tNewfield\tNY\tSchuyler County\tH1\n14805\t36097\tAlpine\tNY\tSchuyler County\tH1\n14863\t36097\tMecklenburg\tNY\tSchuyler County\tH1\n14845\t36097\tHorseheads\tNY\tSchuyler County\tH1\n14891\t36097\tWatkins glen\tNY\tSchuyler County\tH1\n14869\t36097\tOdessa\tNY\tSchuyler County\tH1\n14870\t36097\tPainted post\tNY\tSchuyler County\tH1\n14886\t36097\tTrumansburg\tNY\tSchuyler County\tH1\n14840\t36097\tHammondsport\tNY\tSchuyler County\tH1\n14818\t36097\tBurdett\tNY\tSchuyler County\tH1\n14878\t36097\tRock stream\tNY\tSchuyler County\tH1\n14865\t36097\tMontour falls\tNY\tSchuyler County\tH1\n14841\t36097\tHector\tNY\tSchuyler County\tH1\n14815\t36097\tBradford\tNY\tSchuyler County\tH1\n14864\t36097\tMillport\tNY\tSchuyler County\tH1\n14838\t36097\tErin\tNY\tSchuyler County\tH1\n14893\t36097\tWayne\tNY\tSchuyler County\tH1\n14876\t36097\tReading center\tNY\tSchuyler County\tH1\n14433\t36099\tClyde\tNY\tSeneca County\tH1\n13065\t36099\tFayette\tNY\tSeneca County\tH1\n13148\t36099\tSeneca falls\tNY\tSeneca County\tH1\n13146\t36099\tSavannah\tNY\tSeneca County\tH1\n14541\t36099\tRomulus\tNY\tSeneca County\tH1\n14847\t36099\tInterlaken\tNY\tSeneca County\tH1\n14886\t36099\tTrumansburg\tNY\tSeneca County\tH1\n14588\t36099\tWillard\tNY\tSeneca County\tH1\n14489\t36099\tLyons\tNY\tSeneca County\tH1\n14456\t36099\tGeneva\tNY\tSeneca County\tH1\n14521\t36099\tOvid\tNY\tSeneca County\tH1\n14841\t36099\tHector\tNY\tSeneca County\tH1\n14860\t36099\tLodi\tNY\tSeneca County\tH1\n13165\t36099\tWaterloo\tNY\tSeneca County\tH1\n14532\t36099\tPhelps\tNY\tSeneca County\tH1\n14823\t36101\tCanisteo\tNY\tSteuben County\tH1\n14879\t36101\tSavona\tNY\tSteuben County\tH1\n14512\t36101\tNaples\tNY\tSteuben County\tH1\n14812\t36101\tBeaver dams\tNY\tSteuben County\tH1\n14837\t36101\tDundee\tNY\tSteuben County\tH1\n14843\t36101\tHornell\tNY\tSteuben County\tH1\n14858\t36101\tLindley\tNY\tSteuben County\tH1\n14897\t36101\tWhitesville\tNY\tSteuben County\tH1\n14831\t36101\tCorning\tNY\tSteuben County\tH1\n14885\t36101\tTroupsburg\tNY\tSteuben County\tH1\n14820\t36101\tCameron mills\tNY\tSteuben County\tH1\n14810\t36101\tBath\tNY\tSteuben County\tH1\n14809\t36101\tAvoca\tNY\tSteuben County\tH1\n14806\t36101\tAndover\tNY\tSteuben County\tH1\n14529\t36101\tPerkinsville\tNY\tSteuben County\tH1\n14856\t36101\tKanona\tNY\tSteuben County\tH1\n14437\t36101\tDansville\tNY\tSteuben County\tH1\n14803\t36101\tAlfred station\tNY\tSteuben County\tH1\n14870\t36101\tPainted post\tNY\tSteuben County\tH1\n14873\t36101\tPrattsburgh\tNY\tSteuben County\tH1\n14819\t36101\tCameron\tNY\tSteuben County\tH1\n14855\t36101\tJasper\tNY\tSteuben County\tH1\n14874\t36101\tPulteney\tNY\tSteuben County\tH1\n14418\t36101\tBranchport\tNY\tSteuben County\tH1\n14814\t36101\tBig flats\tNY\tSteuben County\tH1\n14898\t36101\tWoodhull\tNY\tSteuben County\tH1\n14840\t36101\tHammondsport\tNY\tSteuben County\tH1\n14807\t36101\tArkport\tNY\tSteuben County\tH1\n14572\t36101\tWayland\tNY\tSteuben County\tH1\n14821\t36101\tCampbell\tNY\tSteuben County\tH1\n14826\t36101\tCohocton\tNY\tSteuben County\tH1\n14871\t36101\tPine city\tNY\tSteuben County\tH1\n14815\t36101\tBradford\tNY\tSteuben County\tH1\n14877\t36101\tRexville\tNY\tSteuben County\tH1\n14808\t36101\tAtlanta\tNY\tSteuben County\tH1\n14827\t36101\tCoopers plains\tNY\tSteuben County\tH1\n14830\t36101\tCorning\tNY\tSteuben County\tH1\n14801\t36101\tAddison\tNY\tSteuben County\tH1\n14804\t36101\tAlmond\tNY\tSteuben County\tH1\n14839\t36101\tGreenwood\tNY\tSteuben County\tH1\n11729\t36103\tDeer park\tNY\tSuffolk County\tH1\n11726\t36103\tCopiague\tNY\tSuffolk County\tH1\n11788\t36103\tHauppauge\tNY\tSuffolk County\tH1\n11782\t36103\tSayville\tNY\tSuffolk County\tH1\n11791\t36103\tSyosset\tNY\tSuffolk County\tH1\n11955\t36103\tMoriches\tNY\tSuffolk County\tH1\n11972\t36103\tSpeonk\tNY\tSuffolk County\tH1\n11956\t36103\tNew suffolk\tNY\tSuffolk County\tH1\n11973\t36103\tUpton\tNY\tSuffolk County\tH1\n11730\t36103\tEast islip\tNY\tSuffolk County\tH1\n11735\t36103\tFarmingdale\tNY\tSuffolk County\tH1\n11738\t36103\tFarmingville\tNY\tSuffolk County\tH1\n11742\t36103\tHoltsville\tNY\tSuffolk County\tH1\n11764\t36103\tMiller place\tNY\tSuffolk County\tH1\n11789\t36103\tSound beach\tNY\tSuffolk County\tH1\n11784\t36103\tSelden\tNY\tSuffolk County\tH1\n11777\t36103\tPort jefferson\tNY\tSuffolk County\tH1\n11952\t36103\tMattituck\tNY\tSuffolk County\tH1\n11968\t36103\tSouthampton\tNY\tSuffolk County\tH1\n11949\t36103\tManorville\tNY\tSuffolk County\tH1\n11794\t36103\tStony brook\tNY\tSuffolk County\tH1\n11948\t36103\tLaurel\tNY\tSuffolk County\tH1\n11977\t36103\tWesthampton\tNY\tSuffolk County\tH1\n11931\t36103\tAquebogue\tNY\tSuffolk County\tH1\n6390\t36103\tFishers island\tNY\tSuffolk County\tH1\n11704\t36103\tWest babylon\tNY\tSuffolk County\tH1\n11716\t36103\tBohemia\tNY\tSuffolk County\tH1\n11721\t36103\tCenterport\tNY\tSuffolk County\tH1\n11746\t36103\tHuntington station\tNY\tSuffolk County\tH1\n11772\t36103\tPatchogue\tNY\tSuffolk County\tH1\n11758\t36103\tMassapequa\tNY\tSuffolk County\tH1\n11792\t36103\tWading river\tNY\tSuffolk County\tH1\n11953\t36103\tMiddle island\tNY\tSuffolk County\tH1\n11971\t36103\tSouthold\tNY\tSuffolk County\tH1\n11932\t36103\tBridgehampton\tNY\tSuffolk County\tH1\n11975\t36103\tWainscott\tNY\tSuffolk County\tH1\n11739\t36103\tGreat river\tNY\tSuffolk County\tH1\n11970\t36103\tSouth jamesport\tNY\tSuffolk County\tH1\n11713\t36103\tBellport\tNY\tSuffolk County\tH1\n11733\t36103\tEast setauket\tNY\tSuffolk County\tH1\n11740\t36103\tGreenlawn\tNY\tSuffolk County\tH1\n11747\t36103\tMelville\tNY\tSuffolk County\tH1\n11778\t36103\tRocky point\tNY\tSuffolk County\tH1\n11798\t36103\tWyandanch\tNY\tSuffolk County\tH1\n11934\t36103\tCenter moriches\tNY\tSuffolk County\tH1\n11950\t36103\tMastic\tNY\tSuffolk County\tH1\n11967\t36103\tShirley\tNY\tSuffolk County\tH1\n11946\t36103\tHampton bays\tNY\tSuffolk County\tH1\n11978\t36103\tWesthampton beach\tNY\tSuffolk County\tH1\n11958\t36103\tPeconic\tNY\tSuffolk County\tH1\n501\t36103\tHoltsville\tNY\tSuffolk County\tH1\n11701\t36103\tAmityville\tNY\tSuffolk County\tH1\n11703\t36103\tNorth babylon\tNY\tSuffolk County\tH1\n11722\t36103\tCentral islip\tNY\tSuffolk County\tH1\n11731\t36103\tEast northport\tNY\tSuffolk County\tH1\n11751\t36103\tIslip\tNY\tSuffolk County\tH1\n11741\t36103\tHolbrook\tNY\tSuffolk County\tH1\n11757\t36103\tLindenhurst\tNY\tSuffolk County\tH1\n11790\t36103\tStony brook\tNY\tSuffolk County\tH1\n11930\t36103\tAmagansett\tNY\tSuffolk County\tH1\n11980\t36103\tYaphank\tNY\tSuffolk County\tH1\n11717\t36103\tBrentwood\tNY\tSuffolk County\tH1\n11715\t36103\tBlue point\tNY\tSuffolk County\tH1\n11705\t36103\tBayport\tNY\tSuffolk County\tH1\n11743\t36103\tHuntington\tNY\tSuffolk County\tH1\n11755\t36103\tLake grove\tNY\tSuffolk County\tH1\n11754\t36103\tKings park\tNY\tSuffolk County\tH1\n11769\t36103\tOakdale\tNY\tSuffolk County\tH1\n11935\t36103\tCutchogue\tNY\tSuffolk County\tH1\n11795\t36103\tWest islip\tNY\tSuffolk County\tH1\n11933\t36103\tCalverton\tNY\tSuffolk County\tH1\n11796\t36103\tWest sayville\tNY\tSuffolk County\tH1\n11961\t36103\tRidge\tNY\tSuffolk County\tH1\n11951\t36103\tMastic beach\tNY\tSuffolk County\tH1\n11976\t36103\tWater mill\tNY\tSuffolk County\tH1\n11724\t36103\tCold spring harbor\tNY\tSuffolk County\tH1\n11959\t36103\tQuogue\tNY\tSuffolk County\tH1\n11702\t36103\tBabylon\tNY\tSuffolk County\tH1\n11725\t36103\tCommack\tNY\tSuffolk County\tH1\n11727\t36103\tCoram\tNY\tSuffolk County\tH1\n11719\t36103\tBrookhaven\tNY\tSuffolk County\tH1\n11749\t36103\tIslandia\t
